vi "MessageAMC_Create.vi"(0 "reference in":refnum<class "MessageAMC.lvclass">, 5 "error in (no error)":errorcluster, 6 "message queue name":string) -> (14 "amc":refnum<class "MessageAMC.lvclass">, 19 "error out":errorcluster)   [LabVIEW 2019, in "MessageAMC.lvclass"]
doc: "Constructor."
uses:
  MessageAMC.lvclass
  MessageAMC.lvclass/MessageAMC.ctl
  <vilib>/NI/AMC/AMC.lvlib
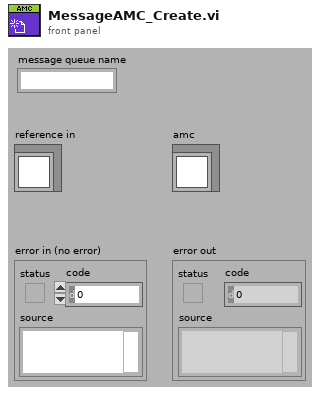
[diagram p1: front panel]
types:
  T1 = typedef "AMC.lvlib/Message Queue.ctl" = refnum<queue>
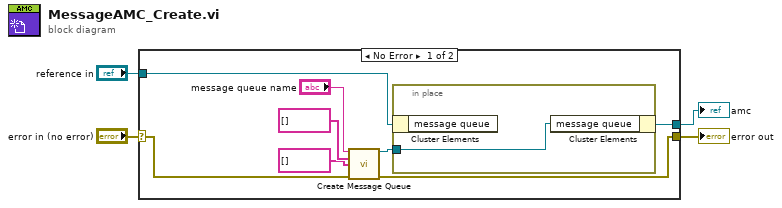
[diagram p0: block diagram]
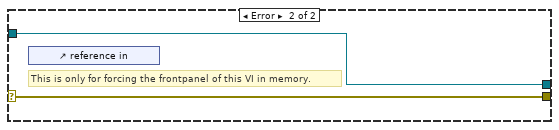
[diagram p2: hidden frame]
diagram:
  n1 = case shown="No Error" "error in (no error)" {
    selector: "error in (no error)" -> [w12 w15]
    tunnel: [w11 w15] -> w3
    tunnel: [w9 w14] -> w1
    tunnel: "reference in" -> [w10 w14]
    frame No Error {
      n2 = call <vilib>:"Create Message Queue.vi"("message queue name"="message queue name", "initial message names"=string[] [], "initial message values"=string[] [], "error in"=w12) -> ("message queue out"=w5:T1, "error out"=w11:errorcluster)  [unwired: 10 in]
      n3 = in-place {
        in-place-border: w5 -> [w13]
        n4 = in-place-cluster #1(w10) -> ()  [unwired: 1 out]
        n5 = in-place-cluster #1("message queue"=w13) -> (w9:refnum<class "MessageAMC.lvclass">)
      }
    }
    frame Error {
      # "This is only for forcing the frontpanel of this VI in memory."
      n6 = control-ref of="reference in"() -> ()  [unwired: 1 out]
    }
  }
  "error out" <- w3
  "amc" <- w1
